vi "limit hit event.vi"(6 "Message handler data":T2, 7 "RT Queues":T1, 11 "Data":variant) -> ()   [LabVIEW 2018]
uses:
  Type Defs/Message loop data.ctl
  Type Defs/FPGA reference.ctl
  Type Defs/RT Status.ctl
  Type Defs/Queues cluster.ctl
  ICL-LabVIEW_General/Message Scheduler/message scheduler.lvclass
  PC/type defs/limitActions.ctl
  Communications loop/create incident - message.vi
  Communications loop/create incident - warning.vi
  Communications loop/create incident - command.vi
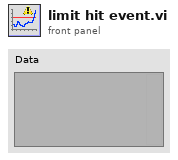
[diagram p1: front panel]
types:
  T1 = typedef "Queues cluster.ctl" = cluster{"RT Message":refnum<queue>, "RT Comms":refnum<queue>, "RT Data":refnum<queue>, "RT FIFO":refnum<queue>, "message scheduler":refnum<class "message scheduler.lvclass">}
  T2 = typedef "Message loop data.ctl" = cluster{"Parameters":cluster{"FPGA Ref":T3, "configID":u32, "activeChannels":cluster{"index":u16, "name":string}[]}, "Variables":cluster{"RT Status":T4, "watchdog":timestamp, "limitsEnabled":bool, "Interlocks":cluster{"gearboxOil":bool, "bearingOil":bool, "gearboxAir":bool}}}
  T3 = typedef "FPGA reference.ctl" = refnum<k20>
  T4 = typedef "RT Status.ctl" = cluster{"Comms loop":bool, "scheduler loop":bool, "data process loop":bool, "FIFO loop":bool, "Command Stream":bool, "Error Stream":bool, "FPGA FIFO":bool, "Data Stream":bool}
  T5 = typedef "limitActions.ctl" = enum16{"stop", "shutdown", "ignore"}
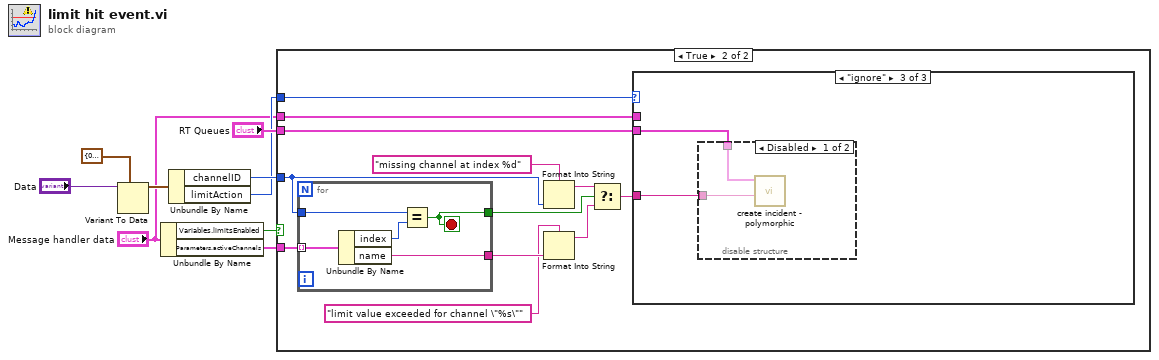
[diagram p0: block diagram]
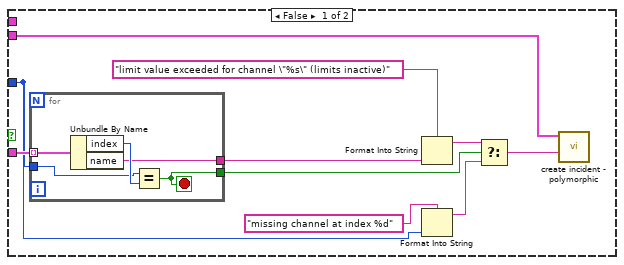
[diagram p2: hidden frame]
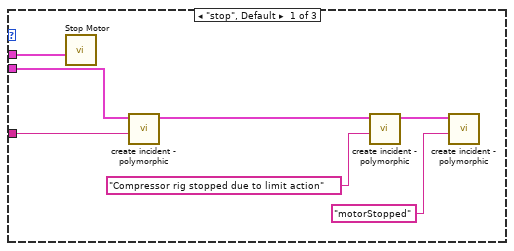
[diagram p3: hidden frame]
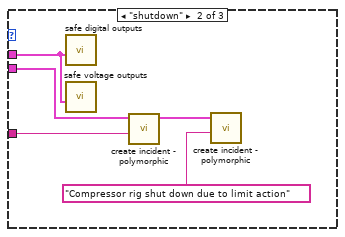
[diagram p4: hidden frame]
diagram:
  n1 = Variant To Data(type=cluster{"channelID":u16, "limitAction":T5} {"channelID"=0, "limitAction"=enum."stop"} ("cluster"), Variant="Data") -> (data=w8:cluster{"channelID":u16, "limitAction":T5})  [unwired: 1 in, 1 out]
  n2 = Unbundle By Name("Message handler data") -> ("Variables.limitsEnabled"=w9:bool, "Parameters.activeChannels"=w4:cluster{"index":u16, "name":string}[])
  n3 = Unbundle By Name(w8) -> ("channelID"=w3:u16, "limitAction"=w2:T5)
  n4 = case shown="True" w9 {
    tunnel: "RT Queues" -> [w19 w27]
    tunnel: w4 -> [w18 w36]
    tunnel: w3 -> [w16 w34]
    tunnel: w2 -> [_ w29]
    tunnel: "Message handler data" -> [_ w26]
    frame False {
      n5 = for {
        tunnel: w18 -> [w24] mode=indexing
        tunnel: w16 -> [w22]
        tunnel: [w21] -> w13
        tunnel: [w20] -> w17
        stop <- w20 stop-if-true
        n6 = Unbundle By Name(w24) -> ("index"=w23:u16, "name"=w21:string)
        n7 = Equal?(x=w22, y=w23) -> (x = y?=w20:bool)
      }
      n8 = Format Into String(format string="limit value exceeded for channel \"%s\" (limits inactive)", w13) -> (resulting string=w12:string)  [unwired: 2 in, 1 out]
      n9 = Format Into String(format string="missing channel at index %d", w16) -> (resulting string=w11:string)  [unwired: 2 in, 1 out]
      n10 = Select(t=w12, s=w17, f=w11) -> (s? t:f=w14:string)
      n11 = call-poly "create incident - polymorphic.vi"("message"=w14, "RT Queues"=w19) -> ()  [unwired: 9 in, 1 out]
    }
    frame True {
      n12 = for {
        tunnel: w36 -> [w57] mode=indexing
        tunnel: w34 -> [w55]
        tunnel: [w54] -> w31
        tunnel: [w53] -> w35
        stop <- w53 stop-if-true
        n13 = Unbundle By Name(w57) -> ("index"=w56:u16, "name"=w54:string)
        n14 = Equal?(x=w55, y=w56) -> (x = y?=w53:bool)
      }
      n15 = Format Into String(format string="missing channel at index %d", w34) -> (resulting string=w32:string)  [unwired: 2 in, 1 out]
      n16 = Format Into String(format string="limit value exceeded for channel \"%s\"", w31) -> (resulting string=w30:string)  [unwired: 2 in, 1 out]
      n17 = Select(t=w32, s=w35, f=w30) -> (s? t:f=w28:string)
      n18 = case shown="\"ignore\"" w29 {
        tunnel: w28 -> [w43 w48 w49]
        tunnel: w27 -> [w42 w47 w50]
        tunnel: w26 -> [w41 w46 _]
        frame "stop", Default {
          n19 = call "Stop Motor.vi"("Message handler data"=w41) -> ()  [unwired: 11 in]
          n20 = call-poly "create incident - polymorphic.vi"("warning description"=w43, "RT Queues"=w42) -> ("RT Queues out"=w40:T1)  [unwired: 9 in]
          n21 = call-poly "create incident - polymorphic.vi"("message"="Compressor rig stopped due to limit action" ("Message"), "RT Queues"=w40) -> ("RT Queues out"=w39:T1)  [unwired: 9 in]
          n22 = call-poly "create incident - polymorphic.vi"("command"="motorStopped" ("Message"), "RT Queues"=w39) -> ()  [unwired: 10 in]
        }
        frame "shutdown" {
          n23 = call "safe digital outputs.vi"("Message handler data"=w46) -> ()  [unwired: 10 in, 1 out]
          n24 = call "safe voltage outputs.vi"("Message handler data"=w46) -> ()  [unwired: 10 in, 1 out]
          n25 = call-poly "create incident - polymorphic.vi"("warning description"=w48, "RT Queues"=w47) -> ("RT Queues out"=w45:T1)  [unwired: 9 in]
          n26 = call-poly "create incident - polymorphic.vi"("message"="Compressor rig shut down due to limit action" ("Message"), "RT Queues"=w45) -> ()  [unwired: 9 in, 1 out]
        }
        frame "ignore" {
          n27 = disable-structure shown="Disabled" {
            disable-tunnel: w50 -> [w52 _]
            disable-tunnel: w49 -> [w51 _]
            frame Disabled {
              n28 = call-poly "create incident - polymorphic.vi"("message"=w51, "RT Queues"=w52) -> ()  [unwired: 9 in, 1 out]
            }
            frame Enabled {
            }
          }
        }
      }
    }
  }
